vi "Initialize Settings.vi"(11 "error in (no error)":errorcluster) -> (3 "Name":string, 4 "Data File Path 2":path, 6 "Address":string, 8 "Comm Port":refnum<visa-resource-name>, 10 "bool":bool, 15 "error out":errorcluster)   [LabVIEW 2012, in "Manager.lvlib" / "Manager.lvclass"]
uses:
  Manager.lvclass
panel:
  in  "Data File Path":path
  in  "Multidrop Number (Unit 0 = 80)":string="€"
  in  "Comm Port":refnum<visa-resource-name>
  in  "Cancel Button":bool
  in  "Name":string
  in  "Button":bool
  # "Enter System Parameters"
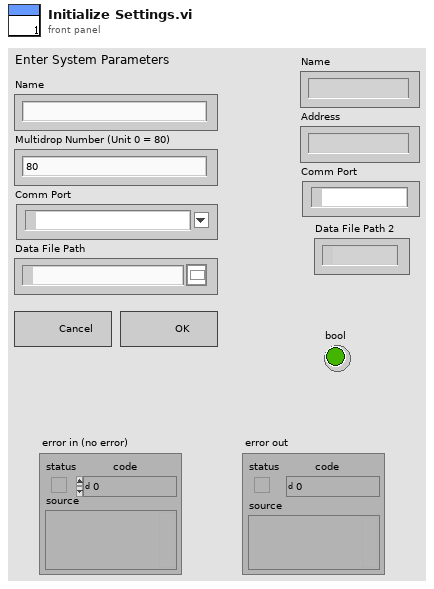
[diagram p1: front panel]
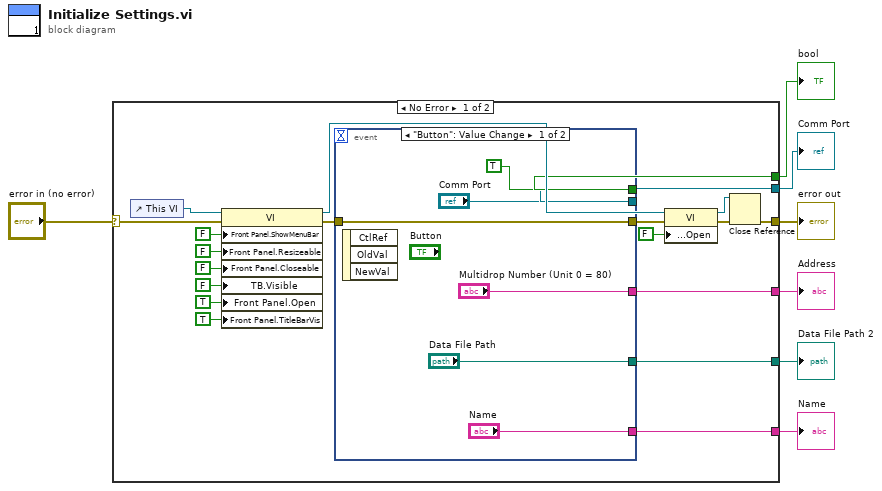
[diagram p0: block diagram]
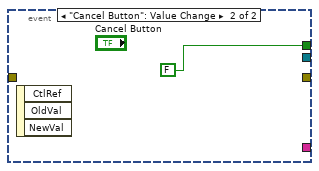
[diagram p2: hidden frame]
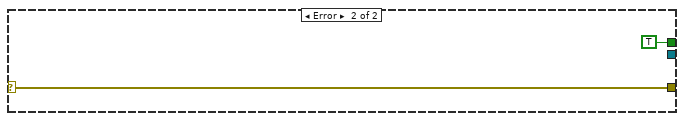
[diagram p3: hidden frame]
diagram:
  n1 = case shown="No Error" "error in (no error)" {
    selector: "error in (no error)" -> [w20 w36]
    tunnel: [w15 w36] -> w6
    tunnel: [w12 TRUE ("Front Panel Window:Open")] -> w5
    tunnel: [w11 _] -> w4
    tunnel: [w10 _] -> w3
    tunnel: [w9 _] -> w2
    tunnel: [w8 _] -> w1
    frame No Error {
      n2 = control-ref of="This VI"() -> (w27:refnum<vi>)
      n3 = property class="VI"(reference=w27, error in=w20, "Front Panel.ShowMenuBar"=FALSE ("Front Panel Window:Show Menu Bar"), "Front Panel.Resizeable"=FALSE ("Front Panel Window:Resizable"), "Front Panel.Closeable"=FALSE ("Front Panel Window:Closeable"), "TB.Visible"=FALSE ("Tool Bar:Visible"), "Front Panel.Open"=TRUE ("Front Panel Window:Open"), "Front Panel.TitleBarVis"=TRUE ("Front Panel Window:Title Bar Visible")) -> (reference out=w14:refnum<vi>, error out=w19:errorcluster)
      n4 = event shown="[0] \"Button\": Value Change" {
        selector: _ -> [_ _]
        dyn-events: _ -> [_ _]
        timeout: _ -> [_ _]
        tunnel: w19 -> [w33 _]
        tunnel: [w33 _] -> w13
        tunnel: [TRUE ("Front Panel Window:Open") FALSE ("Front Panel Window:Open")] -> w12
        tunnel: ["Name" _] -> w11
        tunnel: ["Comm Port" _] -> w10
        tunnel: ["Multidrop Number (Unit 0 = 80)" _] -> w9
        tunnel: ["Data File Path" _] -> w8
        event "Button": Value Change {
          n5 = event-data() -> ()  [unwired: 1 in, 3 out]
        }
        event "Cancel Button": Value Change {
          n6 = event-data() -> ()  [unwired: 1 in, 3 out]
        }
      }
      n7 = property class="VI"(reference=w14, error in=w13, "Front Panel.Open"=FALSE ("Front Panel Window:Open")) -> (reference out=w18:refnum<vi>, error out=w17:errorcluster)
      n8 = Close Reference(reference=w18, error in (no error)=w17) -> (error out=w15:errorcluster)
    }
    frame Error {
    }
  }
  "error out" <- w6
  "bool" <- w5
  "Name" <- w4
  "Comm Port" <- w3
  "Address" <- w2
  "Data File Path 2" <- w1
